vi "Trial time controls.vi"(6 "Elapsed Time (s)":dbl, 9 "Countdown":dbl, 10 "Trial Duration (s)":dbl, 11 "Interruption Times":dbl[](array[numeric])) -> (1 "End of Countdown?":bool, 2 "Trial Complete?":bool, 3 "Countdown":dbl, 4 "Trigger Balloon?":bool)   [LabVIEW 2018, in "CollectionSupport.lvlib"]
uses:
  CollectionSupport.lvlib
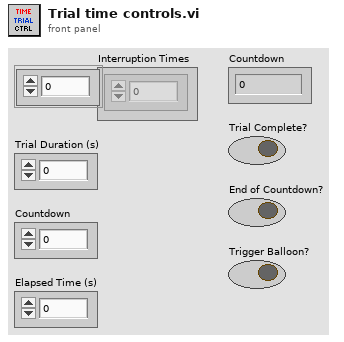
[diagram p1: front panel]
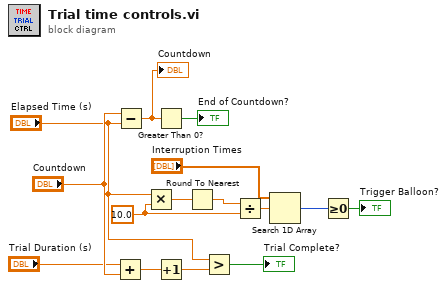
[diagram p0: block diagram]
diagram:
  w2 = 10.0 ("x")
  n1 = Add(x="Trial Duration (s)", y="Countdown") -> (x+y=w10:dbl)
  n2 = Subtract(x="Countdown", y="Elapsed Time (s)") -> (x-y=w5:dbl)
  "Countdown" <- w5
  n3 = Multiply(x="Elapsed Time (s)", y=w2) -> (x*y=w12:dbl)
  n4 = Greater Than 0?(x=w5) -> (x > 0?=→"End of Countdown?":bool)
  n5 = Increment(x=w10) -> (x+1=w9:dbl)
  n6 = Round To Nearest(number=w12) -> (nearest integer value=w13:dbl)
  n7 = Greater?(x="Elapsed Time (s)", y=w9) -> (0:→"Trial Complete?":bool)
  n8 = Divide(x=w13, y=w2) -> (x/y=w14:dbl)
  n9 = Search 1D Array(1D array="Interruption Times", element=w14) -> (index of element=w6:i32)  [unwired: 1 in]
  n10 = Greater Or Equal To 0?(x=w6) -> (x >= 0?=→"Trigger Balloon?":bool)
